vi "Start relative move.vi"(0 "Zaber":T1={"Serial port handle"="", "Axis"="", "Controller #"=0, "Min position"=0.0, "Max position"=0.0, "Min velocity"=0.0, "Max velocity"=0.0, "Firmware"="", "Device ID"=0, "Variable event"=refnum, "Variable ref"=refnum, "Resolution, usteps/step"=0, "Serial port semaphore"=refnum, "Joystick buttons"={"MinDir"=1, "MaxDir"=2, "MedSpeed"=5, "HighSpeed"=6}} {"Joystick buttons"."HighSpeed" min=1 max=25 step=1; "Joystick buttons"."MedSpeed" min=1 max=25 step=1; "Joystick buttons"."MaxDir" min=1 max=25 step=1; "Joystick buttons"."MinDir" min=1 max=25 step=1}, 2 "Distance, mm":dbl, 5 "error in":errorcluster) -> (11 "Start time, ms":u32, 14 "Zaber out":T1={"Serial port handle"="", "Axis"="", "Controller #"=0, "Min position"=0.0, "Max position"=0.0, "Min velocity"=0.0, "Max velocity"=0.0, "Firmware"="", "Device ID"=0, "Variable event"=refnum, "Variable ref"=refnum, "Resolution, usteps/step"=0, "Serial port semaphore"=refnum, "Joystick buttons"={"MinDir"=1, "MaxDir"=2, "MedSpeed"=5, "HighSpeed"=6}} {"Joystick buttons"."HighSpeed" min=1 max=25 step=1; "Joystick buttons"."MedSpeed" min=1 max=25 step=1; "Joystick buttons"."MaxDir" min=1 max=25 step=1; "Joystick buttons"."MinDir" min=1 max=25 step=1}, 19 "error out":errorcluster)   [LabVIEW 2018]
uses:
  Zaber.ctl
  GenericDataEvent/GenericEvent.ctl
  ZaberVariables.ctl
  CommandZaber.ctl
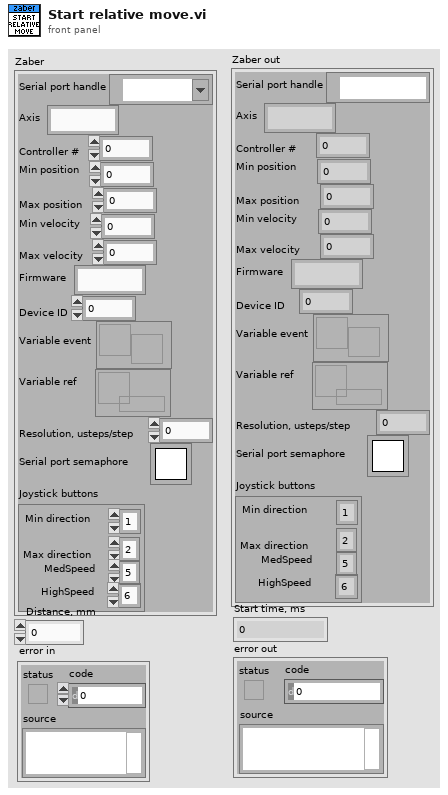
[diagram p1: front panel]
types:
  T1 = typedef "Zaber.ctl" = cluster{"Serial port handle":refnum<visa-resource-name>, "Axis":string, "Controller #":u8, "Min position":dbl, "Max position":dbl, "Min velocity":dbl, "Max velocity":dbl, "Firmware":string, "Device ID":i32, "Variable event":T2, "Variable ref":refnum<data-value>, "Resolution, usteps/step":i32, "Serial port semaphore":T3, "Joystick buttons":cluster{"MinDir":i32, "MaxDir":i32, "MedSpeed":i32, "HighSpeed":i32}}
  T2 = typedef "GenericEvent.ctl" = refnum<user-event>
  T3 = typedef "Semaphore RefNum" = refnum<k1>
  T4 = typedef "CommandZaber.ctl" = cluster{"Command":u8, "Data":i32}
  T5 = typedef "ZaberVariables.ctl" = cluster{"Position":i32, "Speed":i32, "Min soft position":dbl, "Max soft position":dbl, "Accelaration":i32}
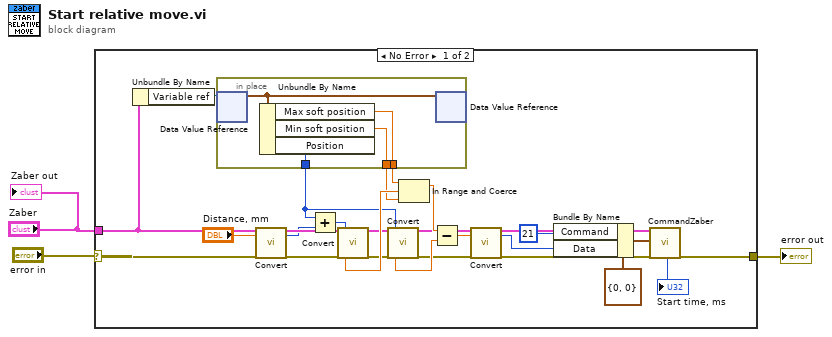
[diagram p0: block diagram]
diagram:
  n1 = case shown="No Error" "error in" {
    selector: "error in" -> [w25 w35]
    tunnel: [w6 w35] -> w2
    tunnel: "Zaber" -> [w24 _]
    frame No Error {
      n2 = Unbundle By Name(w24) -> ("Variable ref"=w22:refnum<data-value>)
      n3 = in-place {
        in-place-border: [w33] -> w14
        in-place-border: [w32] -> w5
        in-place-border: [w31] -> w4
        n4 = in-place-dvr #1(w22) -> (w34:T5)  [unwired: 1 out]
        n5 = Unbundle By Name(w34) -> ("Max soft position"=w32:dbl, "Min soft position"=w31:dbl, "Position"=w33:i32)
        n6 = in-place-dvr #1(w34) -> ()  [unwired: 2 out]
      }
      n7 = call "Convert.vi"("Zaber"=w24, "Position, mm"="Distance, mm", "error in"=w25) -> ("Zaber out"=w20:T1, "Position, usteps"=w19:i32, "error out"=w21:errorcluster)  [unwired: 8 in, 6 out]
      n8 = Add(x=w14, y=w19) -> (x+y=w13:i32)
      n9 = call "Convert.vi"("Zaber"=w20, "error in"=w21, "Position, usteps"=w13) -> ("Position, mm"=w18:dbl, "Zaber out"=w17:T1, "error out"=w16:errorcluster)  [unwired: 8 in, 6 out]
      n10 = call "Convert.vi"("Zaber"=w17, "error in"=w16, "Position, usteps"=w14) -> ("Position, mm"=w15:dbl, "Zaber out"=w10:T1, "error out"=w12:errorcluster)  [unwired: 8 in, 6 out]
      n11 = In Range and Coerce(upper limit=w5, x=w18, lower limit=w4) -> (coerced(x)=w26:dbl)  [unwired: 1 out]
      n12 = Subtract(x=w26, y=w15) -> (x-y=w8:dbl)
      n13 = call "Convert.vi"("Zaber"=w10, "Position, mm"=w8, "error in"=w12) -> ("Zaber out"=w9:T1, "Position, usteps"=w7:i32, "error out"=w11:errorcluster)  [unwired: 8 in, 6 out]
      n14 = Bundle By Name(cluster=T4 {"Command"=0, "Data"=0} ("Command"), "Command"=u8 21, "Data"=w7) -> (w29:T4)
      n15 = call "CommandZaber.vi"("Zaber"=w9, "Command"=w29, "error in"=w11) -> ("Command time, ms"=→"Start time, ms":u32, "error out"=w6:errorcluster)  [unwired: 13 in, 2 out]
    }
    frame Error {
    }
  }
  "error out" <- w2
  "Zaber out" <- "Zaber"
